vi "获取输入频率.vi"(11 "频率配置":i32) -> (3 "频率":dbl[](array[numeric]))   [LabVIEW 2020]
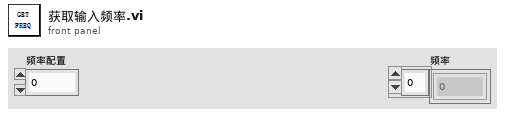
[diagram p1: front panel]
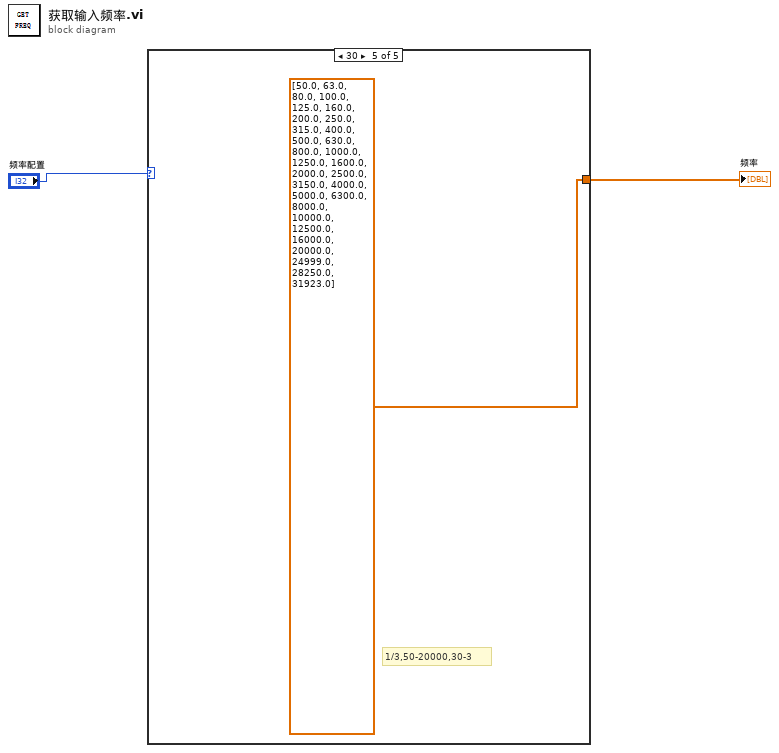
[diagram p0: block diagram]
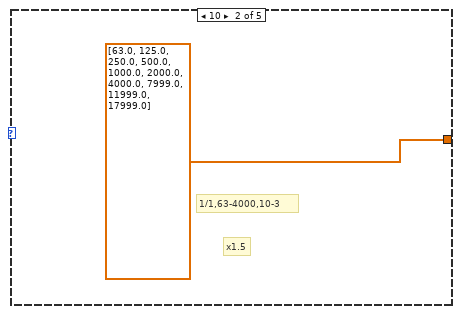
[diagram p3: hidden frame]
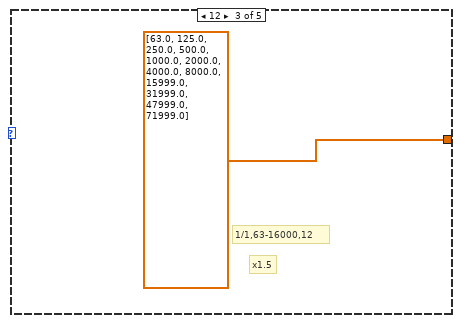
[diagram p4: hidden frame]
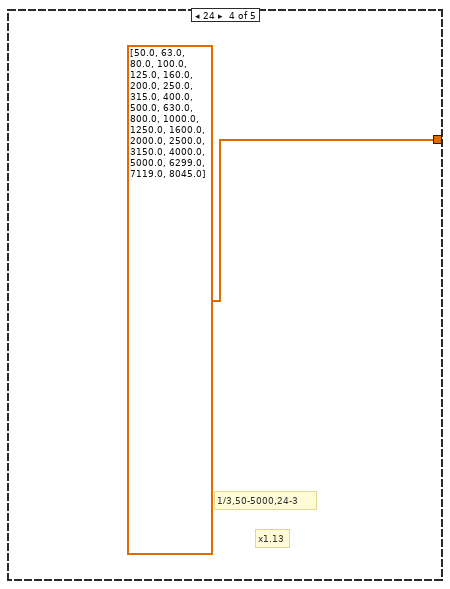
[diagram p5: hidden frame]
diagram:
  n1 = case shown="30" "频率配置" {
    tunnel: [_ dbl[] [63.0, 125.0, 250.0, 500.0, 1000.0, 2000.0, 4000.0, 7999.0, 11999.0, 17999.0] dbl[] [63.0, 125.0, 250.0, 500.0, 1000.0, 2000.0, 4000.0, 8000.0, 15999.0, 31999.0, 47999.0, 71999.0] dbl[] [50.0, 63.0, 80.0, 100.0, 125.0, 160.0, 200.0, 250.0, 315.0, 400.0, 500.0, 630.0, 800.0, 1000.0, 1250.0, 1600.0, 2000.0, 2500.0, 3150.0, 4000.0, 5000.0, 6299.0, 7119.0, 8045.0] dbl[] [50.0, 63.0, 80.0, 100.0, 125.0, 160.0, 200.0, 250.0, 315.0, 400.0, 500.0, 630.0, 800.0, 1000.0, 1250.0, 1600.0, 2000.0, 2500.0, 3150.0, 4000.0, 5000.0, 6300.0, 8000.0, 10000.0, 12500.0, 16000.0, 20000.0, 24999.0, 28250.0, 31923.0]] -> w1
    frame 0, Default {
      # "1/1,63-4000,10"
    }
    frame 10 {
      # "x1.5"
      # "1/1,63-4000,10-3"
    }
    frame 12 {
      # "x1.5"
      # "1/1,63-16000,12"
    }
    frame 24 {
      # "x1.13"
      # "1/3,50-5000,24-3"
    }
    frame 30 {
      # "1/3,50-20000,30-3"
    }
  }
  "频率" <- w1
